vi "Resampling for Power Quality.vi"(0 "data in":waveform(dbl)[](array[waveform]), 2 "reset? (F)":bool, 5 "reference channel index (0)":i32, 9 "system info in":refnum<class "EP System Info.lvclass">, 11 "error in (no error)":errorcluster) -> (4 "resampled data":T1, 10 "system info out":refnum<class "EP System Info.lvclass">, 15 "error out":errorcluster)   [LabVIEW 2014, in "NI_EP_Resample_Host.lvlib"]
doc: "Resamples even-time-spaced voltage and current signals into even-angle-spaced signals. The output signals are synchronous with the line frequency with a constant number of samples per cycle. Use the FPGA Resampling VI if you want to perform resampling on FPGA targets.\n\nThis VI supports measuring single-line and multiple-line systems."
uses:
  <vilib>/addons/Electrical Power/PQ/Resampling/NI_EP_Resample_Host.lvlib
  <vilib>/addons/Electrical Power/PQ/Common/Classes/System Info/EP System Info.lvclass
  <vilib>/addons/Electrical Power/PQ/Resampling/Desktop/subVIs/ep_Resampled Data.ctl
  <vilib>/Analysis/2dsp.llb/Resample (constant to variable, multi-channel).vi
  <vilib>/Analysis/NI_AALPro.lvlib
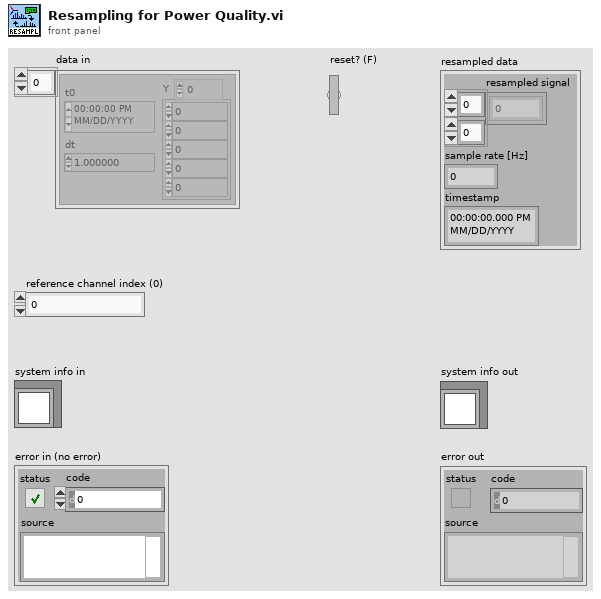
[diagram p1: front panel]
types:
  T1 = typedef "NI_EP_Resample_Host.lvlib/ep_Resampled Data.ctl" = cluster{"resampled signal":dbl[][], "sample rate [Hz]":dbl, "timestamp":timestamp}
  T2 = cluster{"alias rejection (dB)":dbl, "normalized bandwidth":dbl}
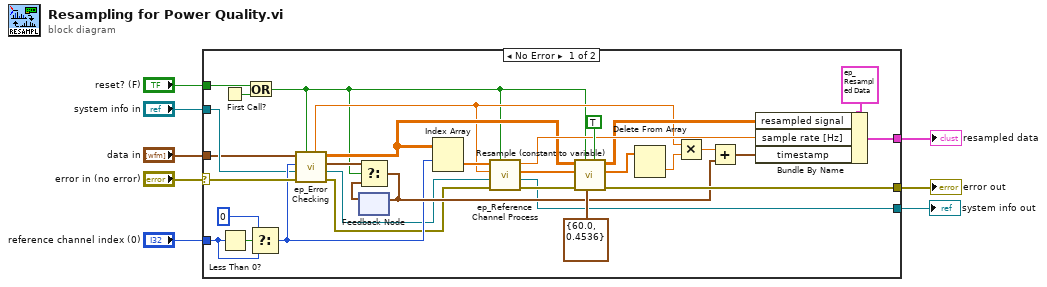
[diagram p0: block diagram]
diagram:
  n1 = case shown="No Error" "error in (no error)" {
    selector: "error in (no error)" -> [w38 w41]
    tunnel: "data in" -> [w21 _]
    tunnel: "reference channel index (0)" -> [w25 _]
    tunnel: "system info in" -> [w22 w42]
    tunnel: [w15 w42] -> w7
    tunnel: [w40 w41] -> w6
    tunnel: "reset? (F)" -> [w37 _]
    tunnel: [w27 _] -> w1
    frame No Error {
      n2 = First Call?() -> (First Call?: T/F=w39:bool)
      n3 = Less Than 0?(x=w25) -> (x < 0?=w26:bool)
      n4 = Or(x=w37, y=w39) -> (x .or. y?=w9:bool)
      n5 = Select(t=0, s=w26, f=w25) -> (s? t:f=w23:i32)
      n6 = call <vilib>:"ep_Error Checking.vi"("reset? (F)"=w9, "error in (no error)"=w38, "system info in"=w22, "reference channel index"=w23, "data"=w21) -> ("error out"=w20:errorcluster, "system info out"=w19:refnum<class "EP System Info.lvclass">, "t0"=w11:timestamp, "signals"=w12:dbl[][], "dt"=w10:dbl)  [unwired: 2 in]
      n7 = feedback #1() -> (w34:timestamp)  [unwired: 1 in]
      n8 = Select(t=w11, s=w9, f=w34) -> (s? t:f=w31:timestamp)
      n9 = feedback-in #1(w31) -> ()
      n10 = Index Array(array=w12, index (row)=w23) -> (element=w16:dbl[])  [unwired: 1 in]
      n11 = call <vilib>:"ep_Reference Channel Process.vi"("reset? (F)"=w9, "error in (no error)"=w20, "system info in"=w19, "dt"=w10, "reference data"=w16) -> ("error out"=w18:errorcluster, "system info out"=w15:refnum<class "EP System Info.lvclass">, "time position"=w17:dbl[], "sampling rate [Hz]"=w14:dbl)  [unwired: 3 in]
      n12 = call-poly <vilib>:"Resample (constant to variable).vi"("anti-aliasing?"=TRUE, "FIR filter specifications"=T2 {"alias rejection (dB)"=60.0, "normalized bandwidth"=0.4536}, "reset?"=w9, "error in (no error)"=w18, "Time"=w17, "X"=w12) -> ("error out"=w40:errorcluster, "Time Stamps"=w33:dbl[], "Y"=w13:dbl[][])  [unwired: 3 in]
      n13 = Delete From Array(array=w33) -> (deleted portion=w32:dbl)  [unwired: 2 in, 1 out]
      n14 = Multiply(x=w10, y=w32) -> (x*y=w30:dbl)
      n15 = Add(x=w30, y=w31) -> (x+y=w29:timestamp)
      n16 = Bundle By Name(cluster=T1 {"resampled signal"=[], "sample rate [Hz]"=0.0, "timestamp"=timestamp(0 s since 1904-01-01)} ("resampled data"), "resampled signal"=w13, "sample rate [Hz]"=w14, "timestamp"=w29) -> (w27:T1)
    }
    frame Error {
    }
  }
  "error out" <- w6
  "system info out" <- w7
  "resampled data" <- w1
